vi "niSE_Configure Channel.vi"(8 "error in":errorcluster, 10 "Channel ID":string, 11 "Handle In":variant) -> (0 "error out":errorcluster {"code" format="%.0x"}, 3 "Handle Out":variant)   [LabVIEW 2015]
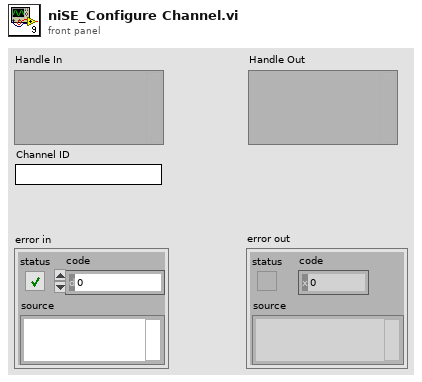
[diagram p1: front panel]
types:
  T1 = typedef "niSE SessionRefnum.ctl" = refnum<k1>
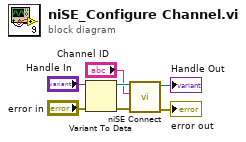
[diagram p0: block diagram]
diagram:
  n1 = Variant To Data(error in="error in", Variant="Handle In") -> (data=w5:T1, error out=w3:errorcluster)  [unwired: 1 in]
  n2 = call <vilib>:"niSE Connect.vi"("error in (no error)"=w3, "Connection Specification (\"\")"="Channel ID", "NISE Session (in)"=w5) -> ("error out"=→"error out":errorcluster, "NISE Session (out)"=→"Handle Out":T1)  [unwired: 7 in]
